vi "Write car state.vi"(8 "error in (no error)":errorcluster, 10 "car state":T1, 11 "Car in":refnum<class "Car.lvclass">) -> (0 "error out":errorcluster, 3 "Car out":refnum<class "Car.lvclass">)   [LabVIEW 2017, in "Car.lvclass"]
uses:
  Car.lvclass
  Car State -- enum.ctl
  Car.lvclass/Car.ctl
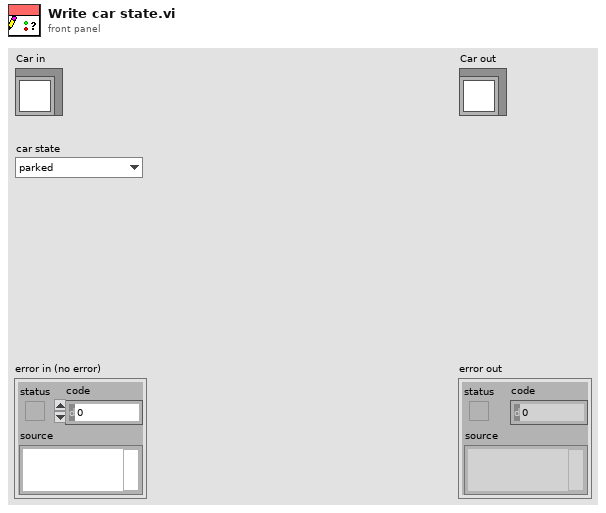
[diagram p1: front panel]
types:
  T1 = typedef "Car.lvclass/Car State -- enum.ctl" = enum16{"parked", "driving"}
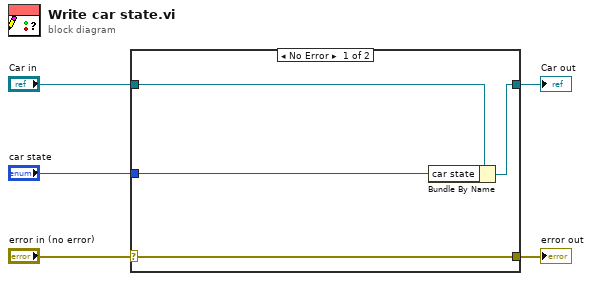
[diagram p0: block diagram]
diagram:
  n1 = case shown="No Error" "error in (no error)" {
    selector: "error in (no error)" -> [w9 w10]
    tunnel: [w9 w10] -> w4
    tunnel: [w7 w11] -> w2
    tunnel: "Car in" -> [w8 w11]
    tunnel: "car state" -> [w6 _]
    frame No Error {
      n2 = Bundle By Name(cluster=w8, "car state"=w6) -> (w7:refnum<class "Car.lvclass">)
    }
    frame Error {
    }
  }
  "error out" <- w4
  "Car out" <- w2
